vi "dual ai kalman step.vi"(6 "AI look-ahead":i16, 8 "y state in":T1, 9 "yval":i16, 10 "x val":i16, 11 "x state in":T1) -> (0 "y state out":T1, 2 "AI values":u32, 3 "x state out":T1)   [LabVIEW 2010]
uses:
  kalman pv state.ctl
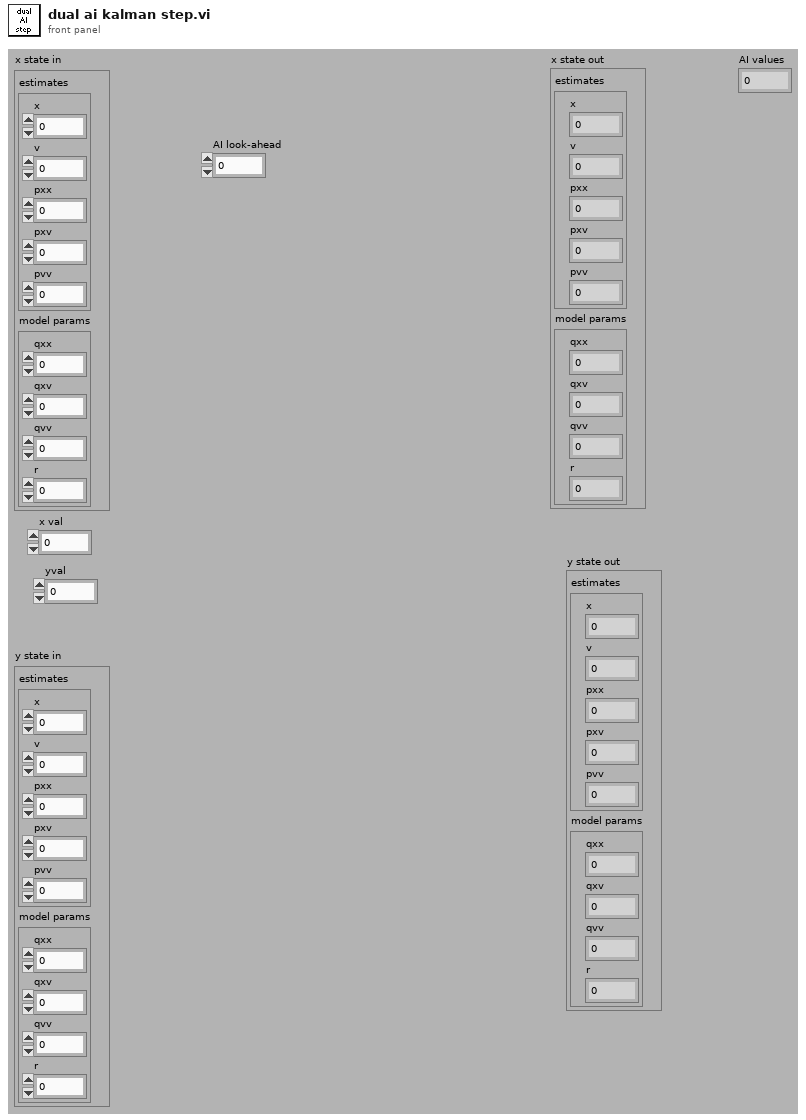
[diagram p1: front panel]
types:
  T1 = typedef "kalman pv state.ctl" = cluster{"estimates":cluster{"x":fxp<+/-,18,16>, "v":fxp<+/-,18,16>, "pxx":u16, "pxv":u16, "pvv":u16}, "model params":cluster{"qxx":u16, "qxv":u16, "qvv":u16, "r":u16}}
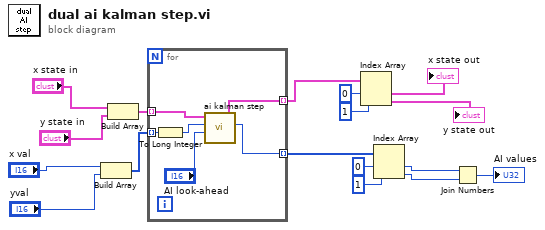
[diagram p0: block diagram]
diagram:
  n1 = Build Array("x val", "yval") -> (w12:i16[])
  n2 = Build Array("x state in", "y state in") -> (w15:T1[])
  n3 = for {
    tunnel: w15 -> [w23] mode=indexing
    tunnel: [w22] -> w11 mode=indexing
    tunnel: w12 -> [w21] mode=indexing
    tunnel: [w18] -> w6 mode=indexing
    n4 = To Long Integer(number=w21) -> (32bit integer=w20:i32)
    n5 = call "ai kalman step.vi"("AI look-ahead"="AI look-ahead", "val in"=w20, "Kalman PV state in"=w23) -> ("estimate"=w18:i16, "kalman pv state out"=w22:T1)  [unwired: 7 in]
  }
  n6 = Index Array(array=w11, index #1=0 ("index"), index #2=1 ("index")) -> (element #1=→"x state out":T1, element #2=→"y state out":T1)
  n7 = Index Array(array=w6, index #1=0 ("index"), index #2=1 ("index")) -> (element #1=w2:i16, element #2=w1:i16)
  n8 = Join Numbers(hi=w2, lo=w1) -> ((hi.lo)=→"AI values":u32)
